vi "_Init Sv.vi"() -> (15 "error out":errorcluster)   [LabVIEW 2019, in "RT_Shared_Variables.lvlib"]
uses:
  Libs/RT_Shared_Variables.lvlib
  TypeDef/State PMG.ctl
  TypeDef/PMG Mode.ctl
  TypeDef/State Engine 2.ctl
  TypeDef/State Engine.ctl
  TypeDef/GUI Setting PMG.ctl
  TypeDef/Needle Valve Settings.ctl
  modbus engine custom/MB_ENGINE_class/Settings.ctl
  TypeDef/Needle Valve Data.ctl
  modbus engine custom/MB_ENGINE_class/Engine State.ctl
  TypeDef/Needle Valve State.ctl
  modbus engine custom/MB_ENGINE_class/Engine Alarms.ctl
  modbus engine custom/MB_ENGINE_class/Limits Status.ctl
  TypeDef/CalibrationData.ctl
  TypeDef/GUI Setting Channel.ctl
  TypeDef/GUI AI Ranges.ctl
  TypeDef/Scale Data.ctl
  TypeDef/AI_Data_Array.ctl
  TypeDef/AI_Data.ctl
  TypeDef/AI Statistics Data.ctl
  TypeDef/error.ctl
  TypeDef/Data Stand.ctl
  TypeDef/Mode.ctl
  TypeDef/ExecuteStepState.ctl
  TypeDef/Direction.ctl
  Modbus_class/STS REG.ctl
  TypeDef/SP_TYPE.ctl
  TypeDef/State 44-1-2.ctl
  FPGA/TypeDef/valveState.ctl
  TypeDef/Setting Stand.ctl
  TypeDef/Pressure Source.ctl
  TypeDef/Setting Pressure PI.ctl
  TypeDef/TCP Connection List.ctl
  <vilib>/NI/Modbus Library/Network Protocol/Network Slave/TCP/Connection.ctl
  modbus engine custom/MB_ENGINE_class/MB_ENGINE.lvclass
  <vilib>/NI/Modbus Library/Network Protocol/Network Slave/TCP/TCP Slave.lvclass
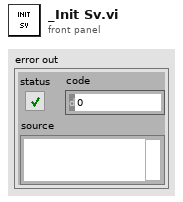
[diagram p1: front panel]
types:
  T1 = typedef "TCP Connection List.ctl" = T2[]
  T2 = typedef "TCP Slave.lvclass/Connection.ctl" = cluster{"Connected?":bool, "IP address":string, "connection error":errorcluster}
  T3 = typedef "Setting Stand.ctl" = cluster{"Pressure Source":T4, "dt pressure down ms":i32, "dP pressure down MPa":dbl, "Haskel":T5, "Pump":T5, "Accuracy [%]":dbl, "Accuracy max [MPa]":dbl, "Accuracy min [MPa]":dbl, "BackPressurVoltage [V]":dbl}
  T4 = typedef "Pressure Source.ctl" = enum16{"Internal", "Modbus", "UDP"}
  T5 = typedef "Setting Pressure PI.ctl" = cluster{"A [MPa/V]":dbl, "P0 [MPa]":dbl}
  T6 = typedef "AI_Data.ctl" = cluster{"Stat Data":T7, "OutOfRangeMax":bool, "OutOfRangeMin":bool, "HIHI":bool, "HI":bool, "LO":bool, "LOLO":bool}
  T7 = typedef "AI Statistics Data.ctl" = cluster{"raw mean":dbl, "scl mean":dbl, "raw mean 1Hz":dbl, "scl mean 1Hz":dbl}
  T8 = typedef "valveState.ctl" = enum16{"Unknown", "Closed", "Opening", "Opened", "Closing"}
  T9 = typedef "Data Stand.ctl" = cluster{"CommCounter":u64, "BeginFilingLevel":dbl, "SP DUT":dbl, "SP CHAMBER":dbl, "Mode":T10, "ExecuteStepState":T11, "Direction":T12, "Direction Filling":T12, "STS":T13, "SP_TYPE_DUT":T14, "SP_TYPE_CHAMBER":T14, "New Step":bool, "BURETE_TIME":u16, "With BURETE":bool, "With Nitro":bool, "State 44-1-2":T15, "Measure leak":bool, "hold":bool}
  T10 = typedef "Mode.ctl" = enum16{"IDLE", "FILLING", "EXECUTE_SP", "DRAIN"}
  T11 = typedef "ExecuteStepState.ctl" = enum16{"Init", "Set: Backpressure ", "Preload: HI", "Set: HI", "Maintenance: HI", "Down: Pressure", "BLOCK"}
  T12 = typedef "Direction.ctl" = enum8{"DUT", "Chamber"}
  T13 = typedef "STS REG.ctl" = cluster{"IDLE":bool, "RYADY":bool, "STEP":bool, "ALARM":bool, "WARNING":bool, "REMOTE":bool, "SP_EXEC_DONE_DUT":bool, "SP_EXEC_DONE_CHAMBER":bool, "FILING_DONE_DUT":bool, "FILING_DONE_CHAMBER":bool, "BURETE_STATE":bool}
  T14 = typedef "SP_TYPE.ctl" = enum16{"ERROR", "ZIRO", "BASE", "SP"}
  T15 = typedef "State 44-1-2.ctl" = enum16{"Init", "Idle", "Wait", "Open 44-1", "Open 44-2", "Close 44-1", "Close 44-2"}
  T16 = typedef "error.ctl" = errorcluster
  T17 = typedef "AI_Data_Array.ctl" = T6[]
  T18 = typedef "CalibrationData.ctl" = cluster{"Channels":T19[], "Scales":T21[]}
  T19 = typedef "GUI Setting Channel.ctl" = cluster{"Name":string, "AI Ranges":T20, "ScaleIndex":u32}
  T20 = typedef "GUI AI Ranges.ctl" = cluster{"HI":bool, "HIHI":bool, "LO":bool, "LOLO":bool, "HIHI VAL":dbl, "HI VAL":dbl, "LO VAL":dbl, "LOLO VAL":dbl, "MAX RAW":dbl, "MIN RAW":dbl, "MAX SCALED":dbl, "MIN SCALED":dbl}
  T21 = typedef "Scale Data.ctl" = cluster{"index":i32, "Name":string, "X":dbl[], "Y":dbl[]}
  T22 = typedef "Needle Valve Data.ctl" = cluster{"Engine State":T23, "StateValveModbus":T24, "Alarms":T25, "RAW":i32, "Angele":dbl, "Step":i32, "Encoder":i32, "Kinematic":T26, "Limits":T27, "EncoderMax":i32, "Counter Max Dont Update":i32, "EncoderMin":i32, "Counter Min Dont Update":i32, "Prepere Counter":i32, "STEP INIT":i32, "offset - Angel":dbl}
  T23 = typedef "MB_ENGINE.lvclass/Engine State.ctl" = u16
  T24 = typedef "Needle Valve State.ctl" = enum16{"STOPED", "CLOSED", "OPENED", "OPENING", "CLOSING", "FULL_CLOSE"}
  T25 = typedef "MB_ENGINE.lvclass/Engine Alarms.ctl" = cluster{"OL":bool, "TF":bool, "STL":bool, "OCP":bool, "CPUV":bool, "UVLO":bool, "SPI_ERROR":bool, "Fault":bool, "OL 2":bool, "TF 2":bool, "STL 2":bool, "OCP 2":bool, "CPUV 2":bool, "UVLO 2":bool, "reserved":bool, "InitDone":bool}
  T26 = typedef "MB_ENGINE.lvclass/Settings.ctl" = cluster{"ACC Steps Per Sec^2":u16, "DEC Steps Per Sec^2":u16, "Min Velosity Step Per Sec":u16, "Max Velosity Step Per Sec":u16, "MicroStep":u16}
  T27 = typedef "MB_ENGINE.lvclass/Limits Status.ctl" = cluster{"Fault 2 Switch":bool, "Fault 1 Switch":bool, "Center(Home)":bool, "Lower Limit":bool, "Upper Limit":bool}
  T28 = typedef "Needle Valve Settings.ctl" = cluster{"average size":i32, "open force":u16, "close force":u16, "open settings":T26, "close settings":T26, "Offset angle":dbl}
  T29 = typedef "GUI Setting PMG.ctl" = cluster{"Temp Turn ON M24":dbl, "Temp Turn OFF M24":dbl, "Temp Open Water M21":dbl, "Temp Close Water M21":dbl, "delta level":dbl, "fililing level %":dbl, "fililing voltage [V]":dbl}
  T30 = typedef "State PMG.ctl" = cluster{"PMG Mode":T31, "M12":T32, "M21":T32, "M24":T32}
  T31 = typedef "PMG Mode.ctl" = enum16{"Idel", "Filling", "Pressure"}
  T32 = typedef "State Engine 2.ctl" = cluster{"EngState":T33, "Active":bool, "Contactor":bool, "CMD":bool, "Automat":bool}
  T33 = typedef "State Engine.ctl" = enum16{"Unknown", "Off", "TupningOn", "On", "TurningOff"}
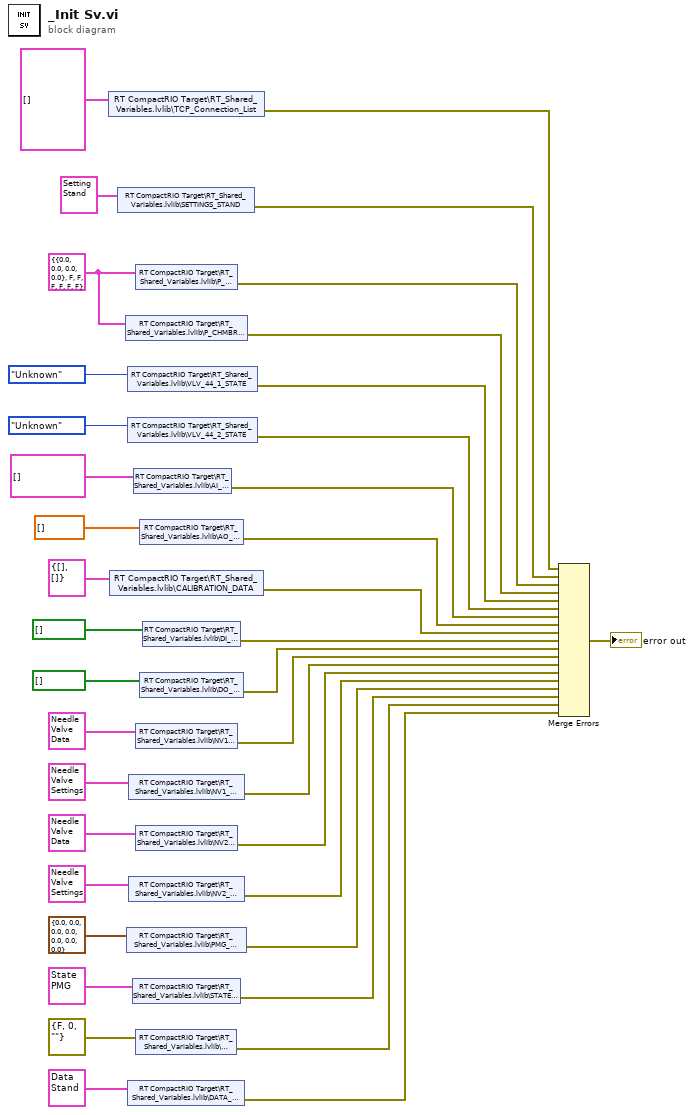
[diagram p0: block diagram]
diagram:
  w5 = T6 {"Stat Data"={"raw mean"=0.0, "scl mean"=0.0, "raw mean 1Hz"=0.0, "scl mean 1Hz"=0.0}, "OutOfRangeMax"=FALSE, "OutOfRangeMin"=FALSE, "HIHI"=FALSE, "HI"=FALSE, "LO"=FALSE, "LOLO"=FALSE} ("P_CHMBR_MB")
  n1 = shared-variable "RT CompactRIO Target\\RT_Shared_Variables.lvlib\\TCP_Connection_List"(T1 [] ("TCP_Connection_List")) -> (error out=w1:errorcluster)  [unwired: 1 in]
  n2 = shared-variable "RT CompactRIO Target\\RT_Shared_Variables.lvlib\\CALIBRATION_DATA"(T18 {"Channels"=[], "Scales"=[]} ("CALIBRATION_DATA")) -> (error out=w26:errorcluster)  [unwired: 1 in]
  n3 = shared-variable "RT CompactRIO Target\\RT_Shared_Variables.lvlib\\SETTINGS_STAND"(T3 {"Pressure Source"=enum."Internal", "dt pressure down ms"=0, "dP pressure down MPa"=0.0, "Haskel"={"A [MPa/V]"=69.0, "P0 [MPa]"=0.0}, "Pump"={"A [MPa/V]"=0.0, "P0 [MPa]"=0.0}, "Accuracy [%]"=0.0, "Accuracy max [MPa]"=0.0, "Accuracy min [MPa]"=0.0, "BackPressurVoltage [V]"=1.0} ("SETTINGS_STAND")) -> (error out=w3:errorcluster)  [unwired: 1 in]
  n4 = shared-variable "RT CompactRIO Target\\RT_Shared_Variables.lvlib\\P_CHMBR_MB"(w5) -> (error out=w7:errorcluster)  [unwired: 1 in]
  n5 = shared-variable "RT CompactRIO Target\\RT_Shared_Variables.lvlib\\PMG_SETTING"(T29 {"Temp Turn ON M24"=0.0, "Temp Turn OFF M24"=0.0, "Temp Open Water M21"=0.0, "Temp Close Water M21"=0.0, "delta level"=0.0, "fililing level %"=0.0, "fililing voltage [V]"=0.0} ("PMG_SETTING")) -> (error out=w19:errorcluster)  [unwired: 1 in]
  n6 = shared-variable "RT CompactRIO Target\\RT_Shared_Variables.lvlib\\VLV_44_1_STATE"(valveState."Unknown" ("VLV_44_1_STATE")) -> (error out=w10:errorcluster)  [unwired: 1 in]
  n7 = shared-variable "RT CompactRIO Target\\RT_Shared_Variables.lvlib\\VLV_44_2_STATE"(valveState."Unknown" ("VLV_44_2_STATE")) -> (error out=w11:errorcluster)  [unwired: 1 in]
  n8 = shared-variable "RT CompactRIO Target\\RT_Shared_Variables.lvlib\\DATA_STAND"(T9 {"CommCounter"=0, "BeginFilingLevel"=0.0, "SP DUT"=0.0, "SP CHAMBER"=0.0, "Mode"=enum."IDLE", "ExecuteStepState"=enum."Init", "Direction"=enum."DUT", "Direction Filling"=enum."DUT", "STS"={"IDLE"=FALSE, "RYADY"=FALSE, "STEP"=FALSE, "ALARM"=FALSE, "WARNING"=FALSE, "REMOTE"=FALSE, "SP_EXEC_DONE_DUT"=FALSE, "SP_EXEC_DONE_CHAMBER"=FALSE, "FILING_DONE_DUT"=FALSE, "FILING_DONE_CHAMBER"=FALSE, "BURETE_STATE"=FALSE}, "SP_TYPE_DUT"=enum."ZIRO", "SP_TYPE_CHAMBER"=enum."ZIRO", "New Step"=FALSE, "BURETE_TIME"=0, "With BURETE"=FALSE, "With Nitro"=FALSE, "State 44-1-2"=enum."Init", "Measure leak"=FALSE, "hold"=FALSE} ("DATA_STAND")) -> (error out=w13:errorcluster)  [unwired: 1 in]
  n9 = shared-variable "RT CompactRIO Target\\RT_Shared_Variables.lvlib\\NV1_SETTING"(T28 {"average size"=0, "open force"=12, "close force"=12, "open settings"={"ACC Steps Per Sec^2"=0, "DEC Steps Per Sec^2"=0, "Min Velosity Step Per Sec"=0, "Max Velosity Step Per Sec"=0, "MicroStep"=0}, "close settings"={"ACC Steps Per Sec^2"=0, "DEC Steps Per Sec^2"=0, "Min Velosity Step Per Sec"=0, "Max Velosity Step Per Sec"=0, "MicroStep"=0}, "Offset angle"=0.0} ("NV_1_SETTING")) -> (error out=w22:errorcluster)  [unwired: 1 in]
  n10 = shared-variable "RT CompactRIO Target\\RT_Shared_Variables.lvlib\\NV2_SETTING"(T28 {"average size"=0, "open force"=12, "close force"=12, "open settings"={"ACC Steps Per Sec^2"=0, "DEC Steps Per Sec^2"=0, "Min Velosity Step Per Sec"=0, "Max Velosity Step Per Sec"=0, "MicroStep"=0}, "close settings"={"ACC Steps Per Sec^2"=0, "DEC Steps Per Sec^2"=0, "Min Velosity Step Per Sec"=0, "Max Velosity Step Per Sec"=0, "MicroStep"=0}, "Offset angle"=0.0} ("NV_2_SETTING")) -> (error out=w20:errorcluster)  [unwired: 1 in]
  n11 = shared-variable "RT CompactRIO Target\\RT_Shared_Variables.lvlib\\STATE_PMG"(T30 {"PMG Mode"=enum."Idel", "M12"={"EngState"=enum."Unknown", "Active"=FALSE, "Contactor"=FALSE, "CMD"=FALSE, "Automat"=FALSE}, "M21"={"EngState"=enum."Unknown", "Active"=FALSE, "Contactor"=FALSE, "CMD"=FALSE, "Automat"=FALSE}, "M24"={"EngState"=enum."Unknown", "Active"=FALSE, "Contactor"=FALSE, "CMD"=FALSE, "Automat"=FALSE}} ("STATE_PMG")) -> (error out=w17:errorcluster)  [unwired: 1 in]
  n12 = shared-variable "RT CompactRIO Target\\RT_Shared_Variables.lvlib\\AI_ARRAY"(T17 [] ("AI_ARRAY")) -> (error out=w28:errorcluster)  [unwired: 1 in]
  n13 = shared-variable "RT CompactRIO Target\\RT_Shared_Variables.lvlib\\P_DUT_MB"(w5) -> (error out=w6:errorcluster)  [unwired: 1 in]
  n14 = shared-variable "RT CompactRIO Target\\RT_Shared_Variables.lvlib\\NV1_DATA"(T22 {"Engine State"=8, "StateValveModbus"=enum."STOPED", "Alarms"={"OL"=FALSE, "TF"=FALSE, "STL"=FALSE, "OCP"=FALSE, "CPUV"=FALSE, "UVLO"=FALSE, "SPI_ERROR"=FALSE, "Fault"=FALSE, "OL 2"=FALSE, "TF 2"=FALSE, "STL 2"=FALSE, "OCP 2"=FALSE, "CPUV 2"=FALSE, "UVLO 2"=FALSE, "reserved"=TRUE, "InitDone"=TRUE}, "RAW"=124110, "Angele"=0.0, "Step"=0, "Encoder"=0, "Kinematic"={"ACC Steps Per Sec^2"=100, "DEC Steps Per Sec^2"=100, "Min Velosity Step Per Sec"=100, "Max Velosity Step Per Sec"=200, "MicroStep"=16}, "Limits"={"Fault 2 Switch"=FALSE, "Fault 1 Switch"=FALSE, "Center(Home)"=FALSE, "Lower Limit"=FALSE, "Upper Limit"=FALSE}, "EncoderMax"=0, "Counter Max Dont Update"=0, "EncoderMin"=0, "Counter Min Dont Update"=0, "Prepere Counter"=0, "STEP INIT"=0, "offset - Angel"=0.0} ("NV_1_DATA")) -> (error out=w23:errorcluster)  [unwired: 1 in]
  n15 = shared-variable "RT CompactRIO Target\\RT_Shared_Variables.lvlib\\NV2_DATA"(T22 {"Engine State"=8, "StateValveModbus"=enum."STOPED", "Alarms"={"OL"=FALSE, "TF"=FALSE, "STL"=FALSE, "OCP"=FALSE, "CPUV"=FALSE, "UVLO"=FALSE, "SPI_ERROR"=FALSE, "Fault"=FALSE, "OL 2"=FALSE, "TF 2"=FALSE, "STL 2"=FALSE, "OCP 2"=FALSE, "CPUV 2"=FALSE, "UVLO 2"=FALSE, "reserved"=TRUE, "InitDone"=TRUE}, "RAW"=124110, "Angele"=0.0, "Step"=0, "Encoder"=0, "Kinematic"={"ACC Steps Per Sec^2"=100, "DEC Steps Per Sec^2"=100, "Min Velosity Step Per Sec"=100, "Max Velosity Step Per Sec"=200, "MicroStep"=16}, "Limits"={"Fault 2 Switch"=FALSE, "Fault 1 Switch"=FALSE, "Center(Home)"=FALSE, "Lower Limit"=FALSE, "Upper Limit"=FALSE}, "EncoderMax"=0, "Counter Max Dont Update"=0, "EncoderMin"=0, "Counter Min Dont Update"=0, "Prepere Counter"=0, "STEP INIT"=0, "offset - Angel"=0.0} ("NV_2_DATA")) -> (error out=w21:errorcluster)  [unwired: 1 in]
  n16 = shared-variable "RT CompactRIO Target\\RT_Shared_Variables.lvlib\\ERROR_BD"(T16 {"status"=FALSE, "code"=0, "source"=""} ("ERROR_BD")) -> (error out=w15:errorcluster)  [unwired: 1 in]
  n17 = shared-variable "RT CompactRIO Target\\RT_Shared_Variables.lvlib\\AO_ARRAY"(dbl[] [] ("AO_ARRAY")) -> (error out=w27:errorcluster)  [unwired: 1 in]
  n18 = shared-variable "RT CompactRIO Target\\RT_Shared_Variables.lvlib\\DO_ARRAY"(bool[] [] ("DO_ARRAY")) -> (error out=w24:errorcluster)  [unwired: 1 in]
  n19 = shared-variable "RT CompactRIO Target\\RT_Shared_Variables.lvlib\\DI_ARRAY"(bool[] [] ("DI_ARRAY")) -> (error out=w25:errorcluster)  [unwired: 1 in]
  n20 = Merge Errors(w1, w3, w6, w7, w10, w11, w28, w27, w26, w25, w24, w23, w22, w21, w20, w19, w17, w15, w13) -> (→"error out":errorcluster)
